vi "Calculate Mean Impulse.vi"(11 "Abstract Fit in":refnum<class "Abstract Fit.lvclass">) -> (3 "Abstract Fit out":refnum<class "Abstract Fit.lvclass">)   [LabVIEW 2013, in "Abstract Fit.lvclass"]
uses:
  Abstract Fit.lvclass
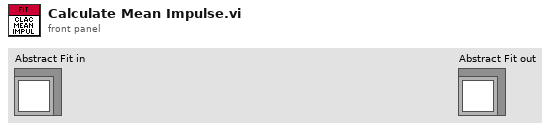
[diagram p1: front panel]
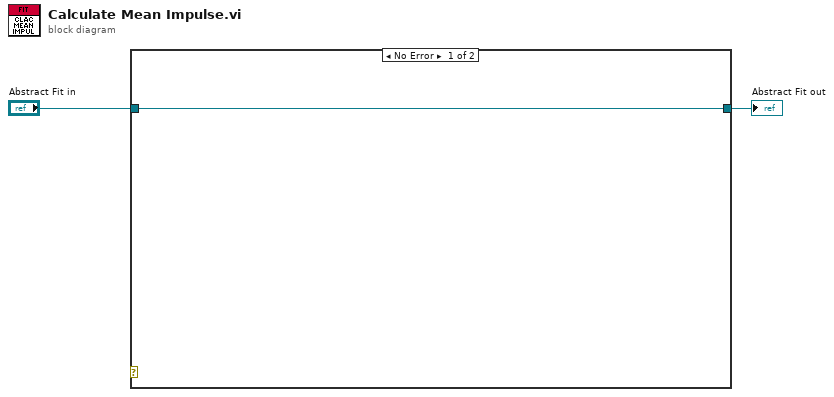
[diagram p0: block diagram]
diagram:
  n1 = case shown="No Error" {
    selector: _ -> [_ w5]
    tunnel: [w3 w4] -> w1
    tunnel: "Abstract Fit in" -> [w3 w4]
    frame No Error {
    }
    frame Error {
    }
  }
  "Abstract Fit out" <- w1
